vi "SDSU_WriteRegister.vi"(8 "error in (no error)":errorcluster, 9 "original Register":T1, 10 "new Register":T1, 11 "fd in":i32) -> (0 "error out":errorcluster, 2 "response":string, 3 "fd out":i32)   [LabVIEW 2016]
uses:
  SDSU_Register.ctl
  SDSU_RegField.ctl
  DBSHAND/private/vis/DatabaseHand_Element_Get(bool).vi
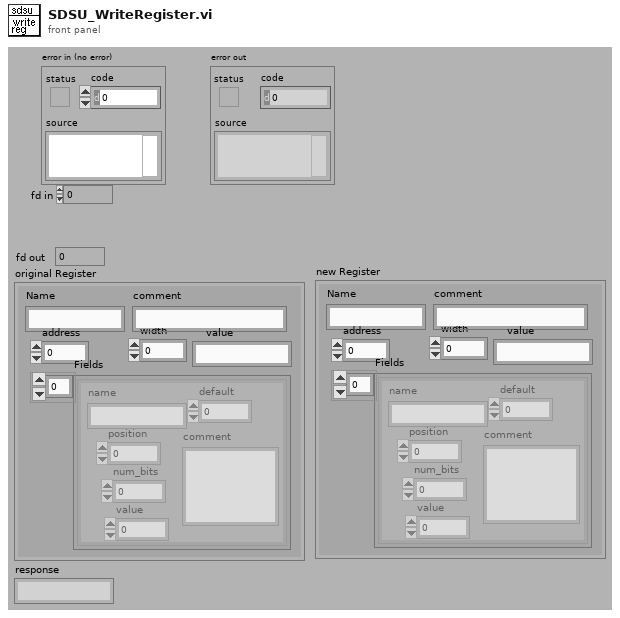
[diagram p1: front panel]
types:
  T1 = typedef "SDSU_Register.ctl" = cluster{"Name":string, "address":i16, "width":i16, "comment":string, "Fields":T2[], "value":string}
  T2 = typedef "SDSU_RegField.ctl" = cluster{"name":string, "position":u16, "num_bits":u16, "default":i16, "comment":string, "value":i32}
  T3 = typedef "DatabaseHand_RefNum.ctl" = refnum<vi>
  T4 = enum16{"READ FROM FILE", "GET ALL", "FIND BY NAME", "SET FIELD VALUE", "CLEAN"}
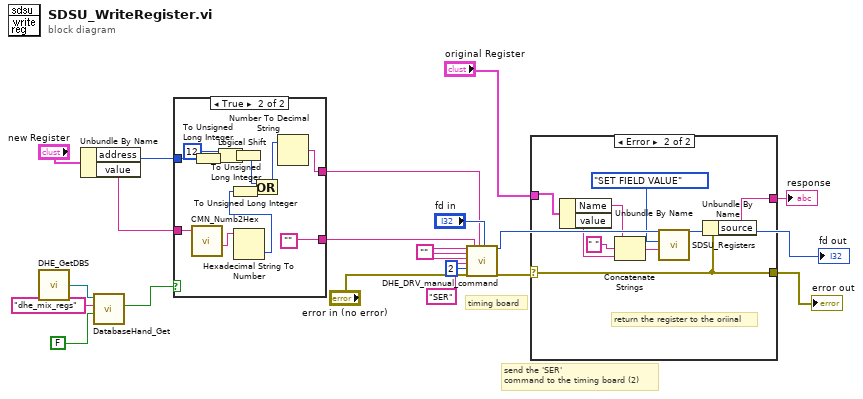
[diagram p0: block diagram]
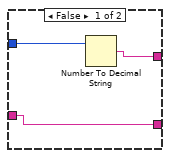
[diagram p2: hidden frame]
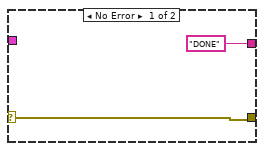
[diagram p3: hidden frame]
diagram:
  w16 = ""
  # "send the 'SER'\ncommand to the timing board (2)"
  # "timing board"
  n1 = call "DHE_GetDBS.vi"() -> ("DHE_DBSRef"=w4:T3)  [unwired: 9 out]
  n2 = Unbundle By Name("new Register") -> ("address"=w8:i16, "value"=w6:string)
  n3 = call-poly "DatabaseHand_Get.vi"("default value"=FALSE, "name"="dhe_mix_regs", "Database RefNum in"=w4) -> ("value"=w1:bool)  [unwired: 2 in, 6 out]
  n4 = case shown="True" w1 {
    tunnel: w8 -> [w22 w34]
    tunnel: [w21 w30] -> w7
    tunnel: w6 -> [w20 w25]
    tunnel: [w20 ""] -> w5
    frame False {
      n5 = Number To Decimal String(number=w22) -> (decimal integer string=w21:string)  [unwired: 1 out]
    }
    frame True {
      n6 = call "CMN_Numb2Hex.vi"("input str"=w25) -> ("output hexa"=w24:string)  [unwired: 10 out]
      n7 = To Unsigned Long Integer(number=w34) -> (unsigned 32bit integer=w28:u32)
      n8 = Logical Shift(y=i8 12, x=w28) -> (x << y=w32:u32)
      n9 = To Unsigned Long Integer(number=w32) -> (unsigned 32bit integer=w27:u32)
      n10 = Hexadecimal String To Number(string=w24) -> (number=w23:u32)  [unwired: 3 out]
      n11 = To Unsigned Long Integer(number=w23) -> (unsigned 32bit integer=w26:u32)
      n12 = Or(x=w27, y=w26) -> (x .or. y?=w31:u32)
      n13 = Number To Decimal String(number=w31) -> (decimal integer string=w30:string)  [unwired: 1 out]
    }
  }
  n14 = call "DHE_DRV_manual_command.vi"("arg3"=w16, "arg4"=w16, "arg5"=w16, "command"="SER", "short board_dest"=i16 2, "error in (no error)"="error in (no error)", "arg2"=w5, "arg1"=w7, "fd"="fd in") -> ("fd"=→"fd out":i32, "error out"=w17:errorcluster)  [unwired: 9 out]
  n15 = case shown="Error" w17 {
    selector: w17 -> [w35 w43]
    tunnel: [w35 w43] -> w11
    tunnel: ["DONE" ("source") w42] -> w9
    tunnel: "original Register" -> [_ w38]
    frame No Error {
    }
    frame Error {
      # "return the register to the oriinal"
      n16 = Unbundle By Name(w38) -> ("Name"=w40:string, "value"=w37:string)
      n17 = Concatenate Strings(w40, " " ("string"), w37) -> (w41:string)
      n18 = call "SDSU_Registers.vi"("argument"=w41, "action"=T4."SET FIELD VALUE") -> ()  [unwired: 2 in, 8 out]
      n19 = Unbundle By Name(w43) -> ("source"=w42:string)
    }
  }
  "error out" <- w11
  "response" <- w9
